vi "Percentage Flow (Set).vi"(6 "ISOBUS address":T3=-1 caption="ISOBUS address (-1)", 8 "error in":errorcluster, 9 "Unit":T1, 10 "Percentage Flow":dbl min=0.0 max=100.0 format="%#.1f", 11 "Mercury Reference In":T5) -> (0 "error out":errorcluster, 2 "Response":T2, 3 "Mercury Reference Out":T5, 4 "Valid?":T4)   [LabVIEW 2015, in "Mercury iXX.lvlib" / "Control Loop.lvlib"]
doc: "Set the percentage of the flow output associated with control loop."
uses:
  Control Loop.lvlib
  Controls/Mercury Reference.ctl
  Controls/Comms Transport Layer.ctl
  private/Controls/Query Dynamic Reference.ctl
  Controls/Is Valid LED.ctl
  Controls/ISOBus Address.ctl
  Controls/Response String.ctl
  Controls/Unit String.ctl
  private/Controls/Command Verbs.ctl
  Mercury iXX.lvlib
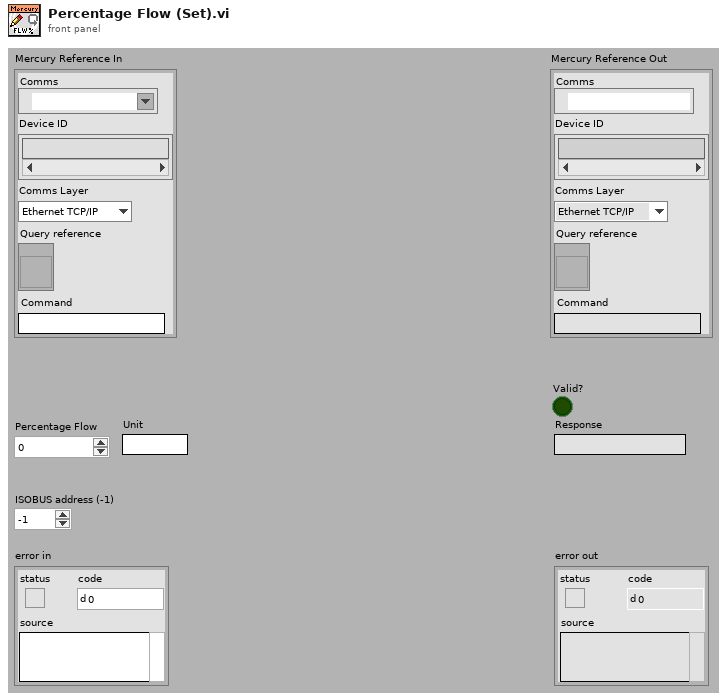
[diagram p1: front panel]
types:
  T1 = typedef "Mercury iXX.lvlib/Unit String.ctl" = string
  T2 = typedef "Mercury iXX.lvlib/Response String.ctl" = string
  T3 = typedef "Mercury iXX.lvlib/ISOBus Address.ctl" = i32
  T4 = typedef "Mercury iXX.lvlib/Is Valid LED.ctl" = bool
  T5 = typedef "Mercury iXX.lvlib/Mercury Reference.ctl" = cluster{"Comms":refnum<visa-resource-name>, "Device ID":string[], "Comms Layer":T6, "Command":string, "Query reference":T7}
  T6 = typedef "Mercury iXX.lvlib/Comms Transport Layer.ctl" = enum16{"Ethernet TCP/IP", "USB", "ISOBus - RS-232", "GPIB"}
  T7 = typedef "Mercury iXX.lvlib/Query Dynamic Reference.ctl" = refnum<vi>
  T8 = typedef "Mercury iXX.lvlib/Command Verbs.ctl" = string
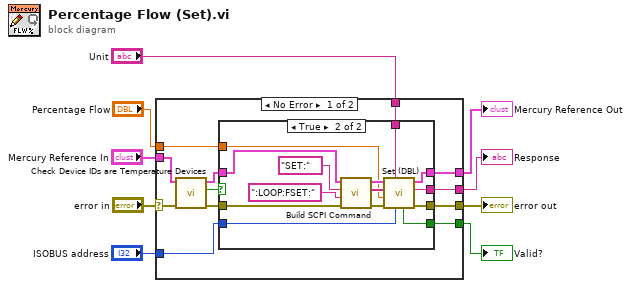
[diagram p0: block diagram]
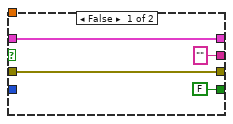
[diagram p2: hidden frame]
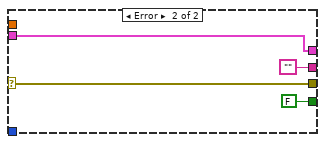
[diagram p3: hidden frame]
diagram:
  n1 = case shown="No Error" "error in" {
    selector: "error in" -> [w16 w42]
    tunnel: "Mercury Reference In" -> [w14 w43]
    tunnel: [w19 w43] -> w5
    tunnel: [w18 w42] -> w2
    tunnel: "ISOBUS address" -> [w20 _]
    tunnel: [w12 ""] -> w4
    tunnel: [w11 FALSE ("Valid?")] -> w3
    tunnel: "Percentage Flow" -> [w21 _]
    tunnel: "Unit" -> [w10 _]
    frame No Error {
      n2 = call "Check Device IDs are Temperature Devices.vi"("error in"=w16, "Mercury Reference In"=w14) -> ("error out"=w15:errorcluster, "Valid?"=w17:bool, "Mercury Reference Out"=w13:T5)  [unwired: 7 out]
      n3 = case shown="True" w17 {
        tunnel: w21 -> [_ w31]
        tunnel: w15 -> [w25 w32]
        tunnel: w20 -> [_ w27]
        tunnel: w13 -> [w24 w35]
        tunnel: [w24 w34] -> w19
        tunnel: [w25 w33] -> w18
        tunnel: [T2 "" ("Response") w29] -> w12
        tunnel: [T4 FALSE ("Valid?") w28] -> w11
        tunnel: w10 -> [_ w26]
        frame False {
        }
        frame True {
          n4 = call "Build SCPI Command.vi"("error in"=w32, "Noun(s)"=":LOOP:FSET:" ("Command"), "Verb"=T8 "SET:", "Mercury Reference In"=w35) -> ("error out"=w39:errorcluster, "SCPI Message(s)"=w38:string[], "Mercury Reference Out"=w37:T5)  [unwired: 5 out]
          n5 = call "Set (DBL).vi"("ISOBUS address"=w27, "Unit"=w26, "error in"=w39, "Command Value (Dbl)"=w31, "SCPI Message(s)"=w38, "Mercury Reference In"=w37) -> ("error out"=w33:errorcluster, "Response"=w29:T2, "Mercury Reference Out"=w34:T5, "Valid?"=w28:T4)  [unwired: 2 out]
        }
      }
    }
    frame Error {
    }
  }
  "Mercury Reference Out" <- w5
  "error out" <- w2
  "Valid?" <- w3
  "Response" <- w4
